vi "PMOD Example(RT).vi"() -> ()   [LabVIEW 2013]
doc: "The continuous acquisition mode tells the FPGA to acquire points indefinitely until a stop command is issued or until an error is encountered (FIFO overflow, module underflow, and so on). \n\nIn this acquisition mode, explicitly call the appropriate rwfm_ConfigTiming VI and set the host application's data buffer to be many times larger than the read size. The examples use a 10X size by default. If the host application's data buffer fills, then the FPGA experiences a FIFO overflow causing the acquisition to stop."
uses:
  <vilib>/rvi/interface/nirviOpenFPGA/nirviOpenFPGA.xnode
  <vilib>/rvi/interface/nirviCloseFPGA/nirviCloseFPGA.xnode
  <vilib>/rvi/interface/nirviMethod/nirviMethod.xnode
  <vilib>/NI_Real-Time Target Support.lvlib
  <vilib>/FPGAPlugInAG/Dynamic/niLvFpga_Reset_Dynamic.vi
  <vilib>/NI/cRIO Wfm/cRIO Wfm.lvlib
  <vilib>/NI/cRIO Wfm/AcqRead(Wfm).vi
  <vilib>/FPGAPlugInAG/Dynamic/niLvFpga_Run_Dynamic.vi
  <vilib>/rvi/interface/nirviReadWriteControl/nirviReadWriteControl.xnode
  <vilib>/Utility/error.llb/Error Cluster From Error Code.vi
  NiFpgaLv.dll
  <vilib>/rvi/interface/Simulation/niFpgaSimulationCallBeginRW.vi
  <vilib>/rvi/errors/niLvFpgaAdjustHostInterfaceError.vi
  <vilib>/measure/NI_MAPro.lvlib
  <vilib>/measure/matone.llb/Extract Single Tone Information 1 Chan.vi
  FPGA Bitfiles/PMOD Driver.lvbitx
  <vilib>/FPGAPlugInAG/sbRIO-9651/niLvFpga_Open_sbRIO-9651.vi
  <vilib>/rvi/interface/common/dynamic/niFpgaDynamicAddResources.vi
  <vilib>/FPGAPlugInAG/Dynamic/niLvFpga_Close_Dynamic.vi
  LucidSPI/Dependencies/cRIO Wfm/_subVIs/RIO Wfm Cust Ctrls/rwfm_ChannelConfig.ctl
  <vilib>/Utility/RT CPU Load.ctl
panel:
  out "Detected Amplitude (V)":dbl format="%.2p"
  in  "Data To ADC":u64=2147483648 format="%.0b"
  in  "SPI PHY Settings":T1={"Divide Value"=20, "Transfer Length (bits)"=32, "CS Asserted Polarity"=FALSE, "Clock Polarity (CPOL)"=FALSE, "Clock Phase (CPHA)"=FALSE, "Lengthen MISO Setup"=FALSE, "Direction Change Bit"=0, "MOSI Starts as Output"=FALSE, "Tristatable MOSI"=FALSE}
  out "Detected Frequency (Hz)":dbl format="%.2p"
  out "Waveform Graph":waveform(dbl)(graph)
  out "CPU loads":T2[](array[typedef])=[{"Total (%)"=29.834964281401128, "Time Critical (%)"=0.0, "Timed Structures (%)"=0.0, "High (%)"=7.025400875853284, "Above Normal (%)"=0.0, "Normal (%)"=22.802136927762042, "Background (%)"=0.007426477785796489, "Idle (%)"=70.16503571859887, "ISR (%)"=0.0}] {"ISR (%)" format="%#.2f"; "Idle (%)" format="%#.2f"; "Background (%)" format="%#.2f"; "Normal (%)" format="%#.2f"; "Above Normal (%)" format="%#.2f"; "High (%)" format="%#.2g"; "Timed Structures (%)" format="%#.2g"; "Time Critical (%)" format="%#.2g"; "Total (%)" format="%#.2g"}
  in  "Sample Rate":dbl=10000.0 caption="Sample Rate (S/s)" format="%#_6p"
  in  "Channel Info":T3=[{"Channel Name"="ai0", "Sensitivity mV_EU"=1000.0, "EU"="V", "dB Ref EU"=1.0}] caption="Channel Name        Scale [mV/EU]        EU           dB Ref [EU]" {"dB Ref EU" format="%#.2p"; "Sensitivity mV_EU" format="%.2f"}
  in  "Samps per Chan":i32=1000 caption="Samples per Channel"
  out "Buffer Backlog":dbl=0.8 caption="RT Buffer Backlog [%]" format="%#.2g"
  in  "stop":bool
  # "Sampling Info"
  # "SPI Settings"
  # "Channel Scaling Info"
  # "1000/Vdd"
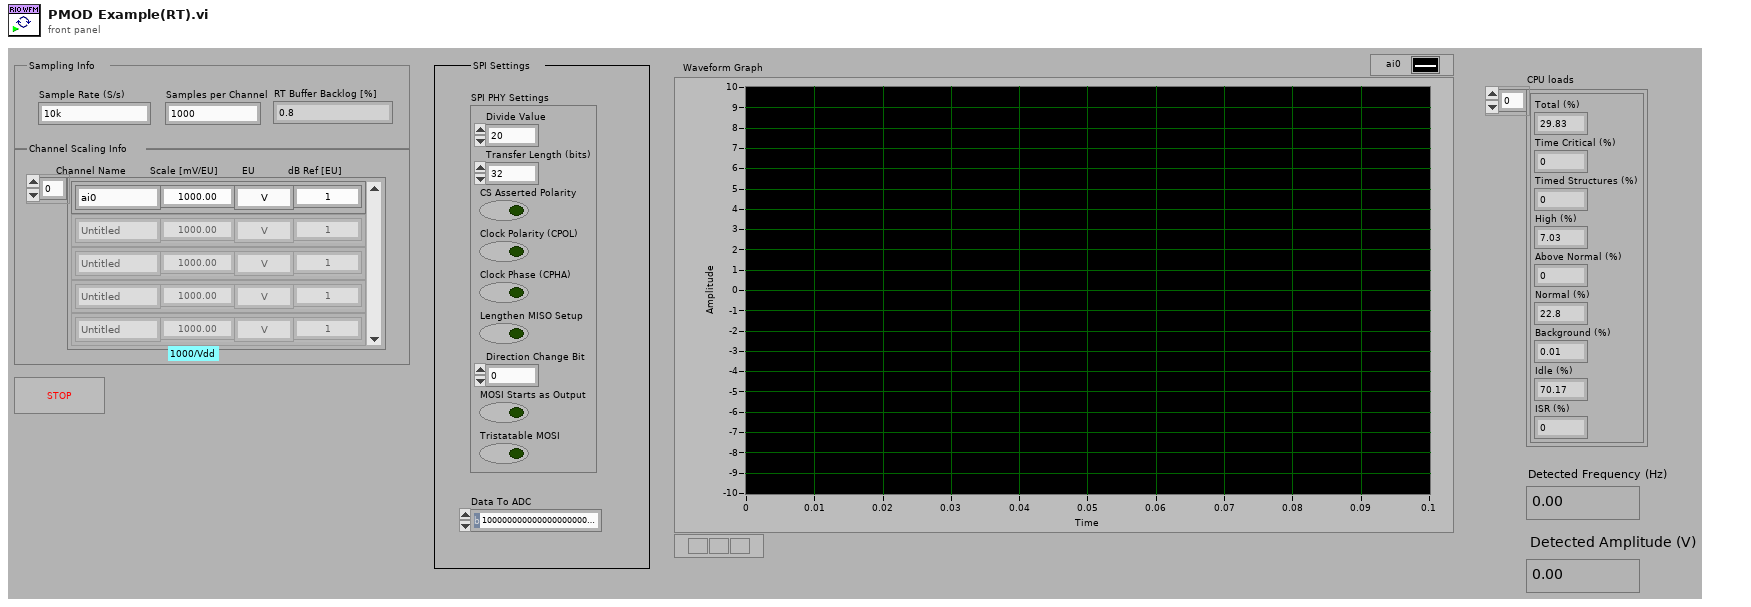
[diagram p1: front panel]
types:
  T1 = cluster{"Divide Value":u8, "Transfer Length (bits)":u8, "CS Asserted Polarity":bool, "Clock Polarity (CPOL)":bool, "Clock Phase (CPHA)":bool, "Lengthen MISO Setup":bool, "Direction Change Bit":u8, "MOSI Starts as Output":bool, "Tristatable MOSI":bool}
  T2 = typedef "NI_Real-Time Target Support.lvlib/RT CPU Load.ctl" = cluster{"Total (%)":dbl, "Time Critical (%)":dbl, "Timed Structures (%)":dbl, "High (%)":dbl, "Above Normal (%)":dbl, "Normal (%)":dbl, "Background (%)":dbl, "Idle (%)":dbl, "ISR (%)":dbl}
  T3 = typedef "rwfm_ChannelConfig.ctl" = cluster{"Channel Name":string, "Sensitivity mV_EU":dbl, "EU":string, "dB Ref EU":dbl}[]
  T4 = typedef "cRIO Wfm.lvlib/SamplingInfo.ctl" = cluster{"Number of Channels":i32, "Actual Samp Rate":dbl, "Chan Name Array":string[], "EU Chan Array":string[], "dB Ref Chan Array":dbl[]}
  T5 = typedef "cRIO Wfm.lvlib/DynamicFPGAref.ctl" = refnum<k20>
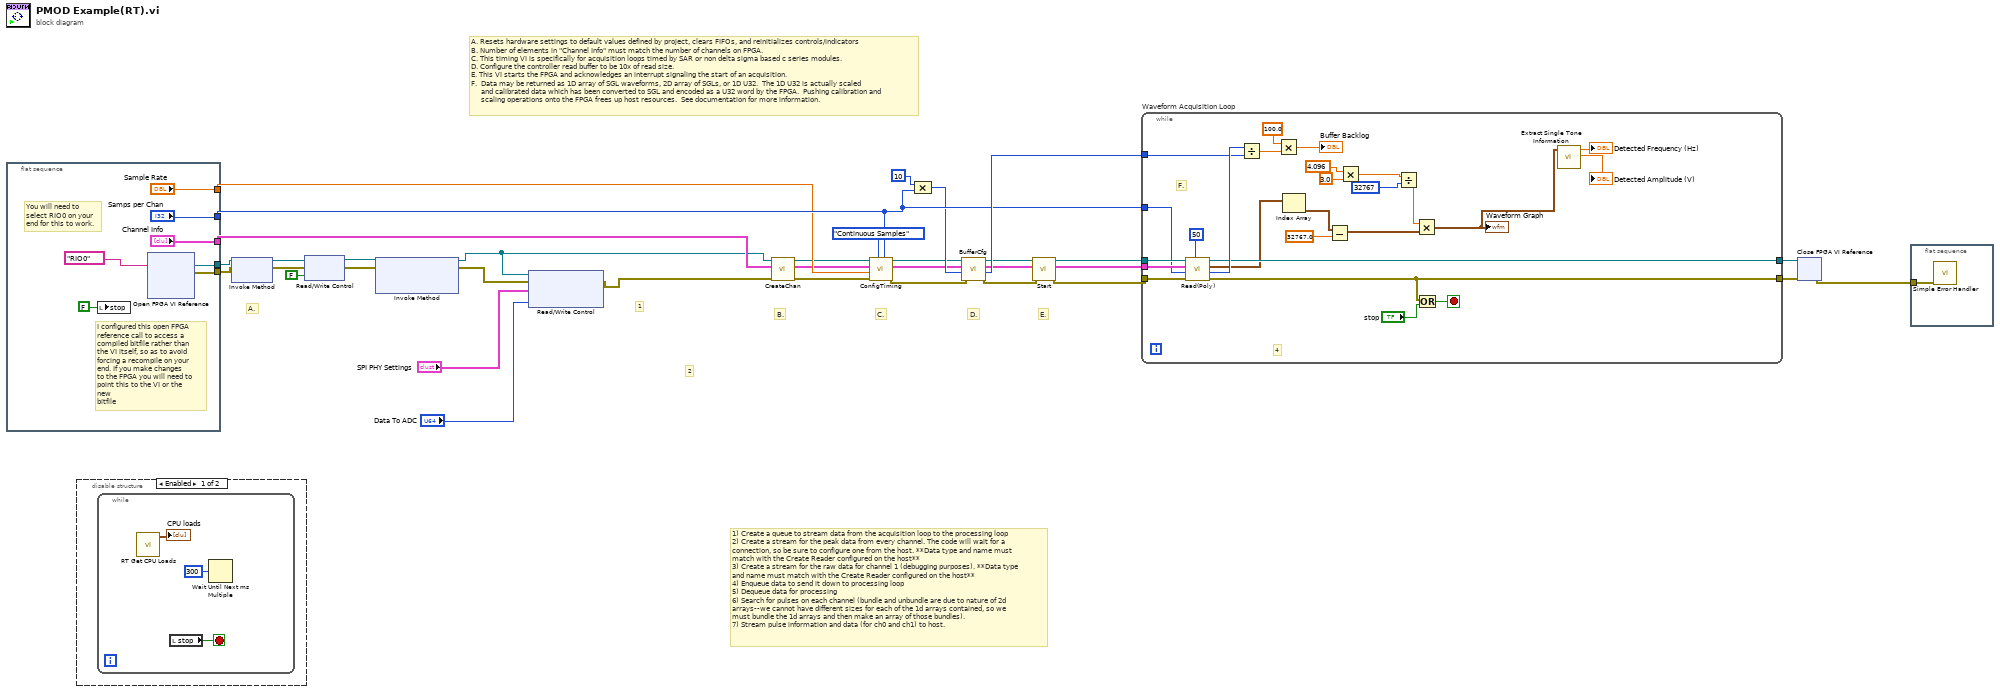
[diagram p0: block diagram]
diagram:
  # "2"
  # "1) Create a queue to stream data from the acquisition loop to the processing loop\n2) Create a stream for the peak data from every channel. The code will wait for a \nconnection, so be sure to configure one from the host. **Data type and name must\nmatch with the Create Reader configured on the host**\n3) Create a stream for the raw data for channel 1 (debugging purposes). **Data type \nand name must match with the Create Reader configured on the host**\n4) Enqueue data to send it down to processing loop\n5) Dequeue data for processing\n6) Search for pulses on each channel (bundle and unbundle are due to nature of 2d\narrays--we cannot have different sizes for each of the 1d arrays contained, so we\nmust bundle the 1d arrays and then make an array of those bundles).\n7) Stream pulse information and data (for ch0 and ch1) to host."
  # "1"
  # "A."
  # "E."
  # "D."
  # "C."
  # "B."
  # "A. Resets hardware settings to default values defined by project, clears FIFOs, and reinitializes controls/indicators\nB. Number of elements in \"Channel Info\" must match the number of channels on FPGA.\nC. This timing VI is specifically for acquisition loops timed by SAR or non delta sigma based c series modules.\nD. Configure the controller read buffer to be 10x of read size.\nE. This VI starts the FPGA and acknowledges an interrupt signaling the start of an acquisition.\nF.  Data may be returned as 1D array of SGL waveforms, 2D array of SGLs, or 1D U32.  The 1D U32 is actually scaled\n     and calibrated data which has been converted to SGL and encoded as a U32 word by the FPGA.  Pushing calibration and\n     scaling operations onto the FPGA frees up host resources.  See documentation for more information."
  n1 = flat-sequence {
    tunnel: ["Samps per Chan"] -> w31
    tunnel: ["Sample Rate"] -> w25
    tunnel: [w38] -> w15
    tunnel: [w37] -> w14
    tunnel: ["Channel Info"] -> w13
    frame #0 {
      # "You will need to\nselect RIO0 on your\nend for this to work."
      # "I configured this open FPGA\nreference call to access a\ncompiled bitfile rather than \nthe VI itself, so as to avoid\nforcing a recompile on your\nend. If you make changes\nto the FPGA you will need to\npoint this to the VI or the new\nbitfile"
      n2 = local write "stop"(FALSE ("stop")) -> ()
      n3 = xnode "Open FPGA VI Reference"("resource name"=tag "RIO0") -> ("FPGA VI Reference Out"=w38:refnum<k20>, "error out"=w37:errorcluster)  [unwired: 1 in]
    }
  }
  n4 = disable-structure shown="Enabled" {
    frame Enabled {
      n5 = while {
        stop <- w43 stop-if-true
        n6 = call <vilib>:"RT Get CPU Loads.vi"() -> ("CPU loads"=→"CPU loads":T2[])  [unwired: 10 in, 1 out]
        n7 = local read "stop"() -> (w43:bool)
        n8 = Wait Until Next ms Multiple(millisecond multiple=u32 300) -> ()  [unwired: 1 out]
      }
    }
    frame Disabled {
    }
  }
  n9 = xnode "Invoke Method"("FPGA VI Reference In"=w15, "error in"=w14) -> ("FPGA VI Reference Out"=w8:refnum<k20>, "error out"=w7:errorcluster)
  n10 = xnode "Read/Write Control"("FPGA VI Reference In"=w8, "error in"=w7, "Debug"=FALSE) -> ("FPGA VI Reference Out"=w6:refnum<k20>, "error out"=w5:errorcluster)
  n11 = xnode "Invoke Method"("FPGA VI Reference In"=w6, "error in"=w5) -> ("FPGA VI Reference Out"=w9:refnum<k20>, "error out"=w11:errorcluster)  [unwired: 1 in]
  n12 = xnode "Read/Write Control"("FPGA VI Reference In"=w9, "error in"=w11, "SPI PHY Settings"="SPI PHY Settings", "Data To ADC"="Data To ADC") -> ("error out"=w10:errorcluster)  [unwired: 1 out]
  n13 = call <vilib>:"CreateChan.vi"("error in"=w10, "Channel Info"=w13, "Dynamic FPGA Ref"=w9) -> ("error out"=w19:errorcluster, "Sampling Info"=w16:T4, "Dynamic FPGA Ref Out"=w20:T5)  [unwired: 6 in]
  n14 = call <vilib>:"ConfigTiming.vi"("Samples per Channel"=w31, "Sample Mode"=enum16{"Finite Samples", "Continuous Samples"}."Continuous Samples", "error in"=w19, "Sample Rate"=w25, "Sampling Info In"=w16, "Dynamic FPGA Ref"=w20) -> ("error out"=w23:errorcluster, "Sampling Info Out"=w18:T4, "Dynamic FPGA Ref Out"=w24:T5)  [unwired: 2 in, 1 out]
  n15 = Compound Arithmetic op=MULTIPLY(10 ("value"), w31) -> (w26:i32)
  n16 = call <vilib>:"BufferCfg.vi"("error in"=w23, "Buffer Size [Samps per Chan]"=w26, "Sampling Info In"=w18, "Dynamic FPGA Ref"=w24) -> ("error out"=w21:errorcluster, "Buffer Size [Total Samples]"=w32:u32, "Sampling Info Out"=w17:T4, "Dynamic FPGA Ref Out"=w22:T5)  [unwired: 4 in]
  n17 = call <vilib>:"Start.vi"("error in"=w21, "Sampling Info In"=w17, "Dynamic FPGA Ref"=w22) -> ("error out"=w30:errorcluster, "Sampling Info Out"=w33:T4, "Dynamic FPGA Ref Out"=w29:T5)  [unwired: 6 in]
  n18 = while "Waveform Acquisition Loop" {
    tunnel: w29 -> [w62]
    tunnel: w30 -> [w69]
    tunnel: [w59] -> w34
    tunnel: w33 -> [w68]
    tunnel: w32 -> [w66]
    tunnel: w31 -> [w61]
    tunnel: [w56] -> w3
    stop <- w70 stop-if-true
    # "4"
    # "F."
    n19 = call-poly <vilib>:"Read(Poly).vi"("Poll Time (ms)"=u32 50, "error in"=w69, "Samps Read per Chan"=w61, "Sampling Info"=w68, "Dynamic FPGA Ref"=w62) -> ("error out"=w56:errorcluster, "Samples Remaining"=w67:u32, "Wfm Data"=w57:waveform(sgl)[], "Dynamic FPGA Ref Out"=w59:T5)  [unwired: 3 in]
    n20 = Divide(x=w67, y=w66) -> (x/y=w65:dbl)
    n21 = Multiply(x=100.0, y=w65) -> (x*y=→"Buffer Backlog":dbl)
    n22 = Index Array(array=w57) -> (element=w47:waveform(sgl))  [unwired: 1 in]
    n23 = Subtract(x=w47, y=32767.0 ("x")) -> (x-y=w54:waveform(dbl))
    n24 = Multiply(x=4.096, y=3.0) -> (x*y=w49:dbl)
    n25 = Divide(x=w49, y=32767) -> (x/y=w52:dbl)
    n26 = Multiply(x=w52, y=w54) -> (x*y=w46:waveform(dbl))
    "Waveform Graph" <- w46
    n27 = Or(x=w56, y="stop") -> (x .or. y?=w70:bool)
    n28 = call-poly <vilib>:"Extract Single Tone Information.vi"("time signal in"=w46) -> ("detected amplitude"=→"Detected Amplitude (V)":dbl, "detected frequency"=→"Detected Frequency (Hz)":dbl)  [unwired: 5 in, 4 out]
  }
  n29 = xnode "Close FPGA VI Reference"("FPGA VI Reference In"=w34, "error in"=w3) -> ("error out"=w12:errorcluster)
  n30 = flat-sequence {
    tunnel: w12 -> [w71]
    frame #0 {
      n31 = call <vilib>:"Simple Error Handler.vi"("error in (no error)"=w71) -> ()  [unwired: 1 in, 8 out]
    }
  }
